vi "Turn.vi"(10 "Right Setpoint":dbl, 11 "Left Setpoint":dbl) -> ()   [LabVIEW 2019]
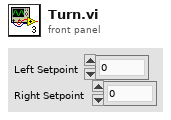
[diagram p1: front panel]
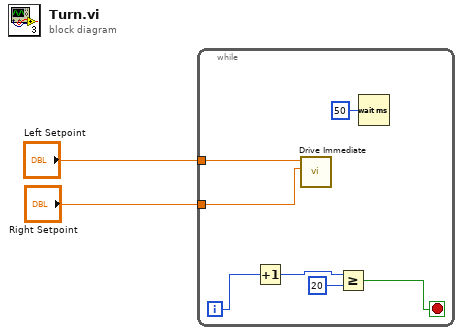
[diagram p0: block diagram]
diagram:
  n1 = while {
    tunnel: "Left Setpoint" -> [w4]
    tunnel: "Right Setpoint" -> [w3]
    i -> [w8]
    stop <- w6 stop-if-true
    n2 = Increment(x=w8) -> (x+1=w7:i32)
    n3 = call "Drive Immediate.vi"("Right Setpoint"=w3, "Left Setpoint"=w4) -> ()  [unwired: 9 in, 1 out]
    n4 = Greater Or Equal?(x=w7, y=20) -> (x >= y?=w6:bool)
    n5 = Wait (ms)(milliseconds to wait=u32 50) -> ()  [unwired: 1 out]
  }
